vi "Insert Soak Step.vi"(0 "VISA resource name":refnum<visa-resource-name>, 1 "Current Step Number (1)":i16=1, 2 "Wait For Event Inputs (0; 0; 0; 0)":u16[](array[ring])=[0, 0, 0, 0] items=["Don't Wait", "Wait For Off", "Wait For On"], 3 "Wait For Analog Inputs (0; 0; 0)":u16[](array[ring])=[0, 0, 0] items=["Don't Wait", "Wait For Analog Input"], 4 "Analog Input Values (0.0; 0.0; 0.0)":dbl[](array[numeric])=[32.0, 32.0, 32.0] format="%.2f", 5 "error in (no error)":errorcluster {"code" format="%.0x"}, 6 "Unit Address (1)":i16=1, 7 "Event Outputs (0; 0; 0; 0; 0; 0; 0; 0)":u16[](array[ring])=[0, 0, 0, 0, 0, 0, 0, 0] items=["Off", "On"], 8 "Wait For Event (0: No)":u16(ring) items=["No", "Yes"], 9 "Time (0; 0; 1)":i16[](array[numeric])=[0, 0, 1], 10 "Channel 1 Guarantee Soak (F: Off)":bool, 11 "Channel 1 PID Set (1)":u16=1, 12 "Channel 2 Guarantee Soak (F: Off)":bool, 13 "Channel 2 PID Set (6)":u16=6) -> (14 "VISA resource name out":refnum<visa-resource-name>, 19 "error out":errorcluster {"code" format="%.0x"})   [LabVIEW 2010]
doc: "This VI inserts Soak Step."
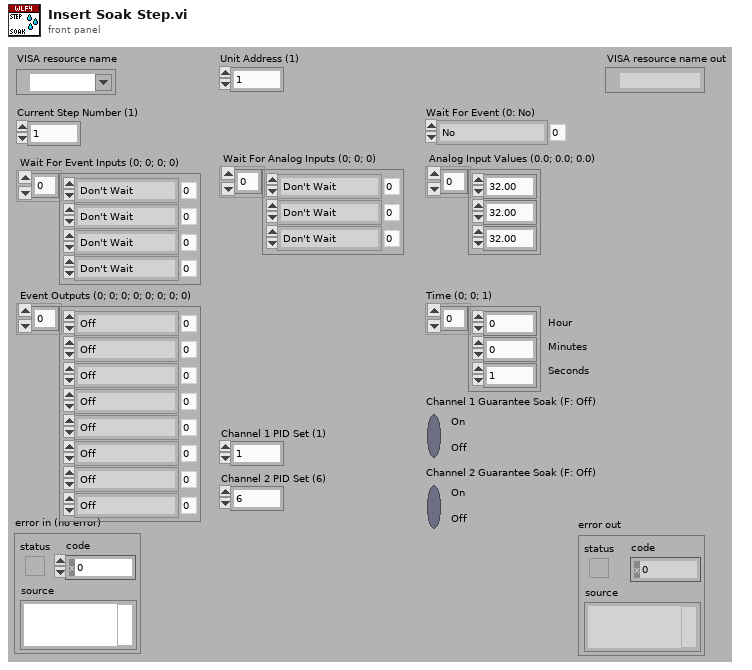
[diagram p1: front panel]
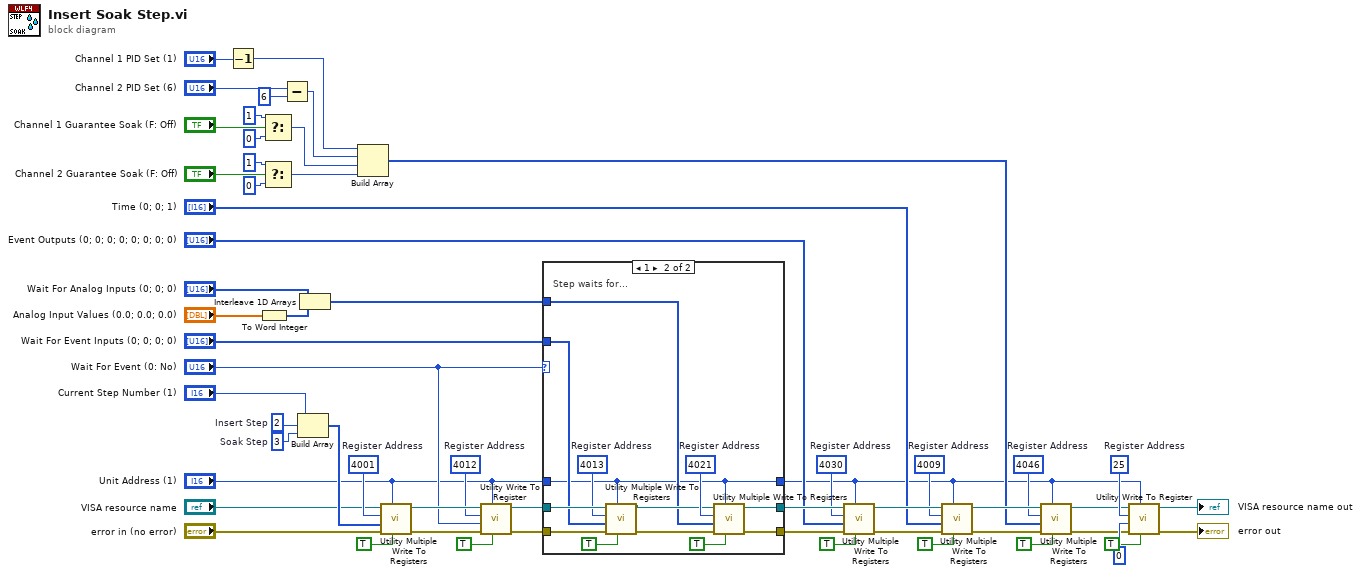
[diagram p0: block diagram]
diagram:
  w18 = u16 4046  # Register Address
  w21 = u16 4009  # Register Address
  w22 = 3  # Soak Step
  w29 = u16 25  # Register Address
  w37 = u16 4030  # Register Address
  w49 = u16 4012  # Register Address
  w55 = u16 2  # Insert Step
  w57 = u16 4001  # Register Address
  n1 = Decrement(x="Channel 1 PID Set (1)") -> (x-1=w7:u16)
  n2 = To Word Integer(number="Analog Input Values (0.0; 0.0; 0.0)") -> (16bit integer=w42:i16[])
  n3 = Select(t=1, s="Channel 1 Guarantee Soak (F: Off)", f=0) -> (s? t:f=w16:i32)
  n4 = Select(t=1, s="Channel 2 Guarantee Soak (F: Off)", f=0) -> (s? t:f=w17:i32)
  n5 = Subtract(x="Channel 2 PID Set (6)", y=u16 6) -> (x-y=w8:u16)
  n6 = Build Array("Current Step Number (1)", w55, w22) -> (w56:i32[])
  n7 = Interleave 1D Arrays("Wait For Analog Inputs (0; 0; 0)", w42) -> (w40:u16[])
  n8 = Build Array(w7, w8, w16, w17) -> (w15:i32[])
  n9 = call "Utility Multiple Write To Registers.vi"("Direct Action?"=TRUE, "Unit Address (1)"="Unit Address (1)", "error in (no error)"="error in (no error)", "Array Of Data"=w56, "Register Address (0)"=w57, "VISA resource name"="VISA resource name") -> ("error out"=w51:errorcluster, "VISA resource name out"=w50:refnum<visa-resource-name>)  [unwired: 4 in]
  n10 = call "Utility Write To Register.vi"("Direct Action?"=TRUE, "Unit Address (1)"="Unit Address (1)", "error in (no error)"=w51, "Data (0)"="Wait For Event (0: No)", "Register Address (0)"=w49, "VISA resource name"=w50) -> ("error out"=w47:errorcluster, "VISA resource name out"=w48:refnum<visa-resource-name>)  [unwired: 4 in]
  n11 = case shown="1" "Wait For Event (0: No)" {
    tunnel: w48 -> [w60 w72]
    tunnel: w47 -> [w59 w73]
    tunnel: [w59 w65] -> w39
    tunnel: [w60 w64] -> w38
    tunnel: "Unit Address (1)" -> [w58 w63]
    tunnel: [w58 w63] -> w14
    tunnel: "Wait For Event Inputs (0; 0; 0; 0)" -> [_ w70]
    tunnel: w40 -> [_ w66]
    frame 0, Default {
      # "Step does not wait"
    }
    frame 1 {
      w69 = u16 4021  # Register Address
      w71 = u16 4013  # Register Address
      # "Step waits for..."
      n12 = call "Utility Multiple Write To Registers.vi"("Direct Action?"=TRUE, "Unit Address (1)"=w63, "error in (no error)"=w73, "Array Of Data"=w70, "Register Address (0)"=w71, "VISA resource name"=w72) -> ("error out"=w68:errorcluster, "VISA resource name out"=w67:refnum<visa-resource-name>)  [unwired: 4 in]
      n13 = call "Utility Multiple Write To Registers.vi"("Direct Action?"=TRUE, "Unit Address (1)"=w63, "error in (no error)"=w68, "Array Of Data"=w66, "Register Address (0)"=w69, "VISA resource name"=w67) -> ("error out"=w65:errorcluster, "VISA resource name out"=w64:refnum<visa-resource-name>)  [unwired: 4 in]
    }
  }
  n14 = call "Utility Multiple Write To Registers.vi"("Direct Action?"=TRUE, "Unit Address (1)"=w14, "error in (no error)"=w39, "Array Of Data"="Event Outputs (0; 0; 0; 0; 0; 0; 0; 0)", "Register Address (0)"=w37, "VISA resource name"=w38) -> ("error out"=w32:errorcluster, "VISA resource name out"=w31:refnum<visa-resource-name>)  [unwired: 4 in]
  n15 = call "Utility Multiple Write To Registers.vi"("Direct Action?"=TRUE, "Unit Address (1)"=w14, "error in (no error)"=w32, "Array Of Data"="Time (0; 0; 1)", "Register Address (0)"=w21, "VISA resource name"=w31) -> ("error out"=w19:errorcluster, "VISA resource name out"=w20:refnum<visa-resource-name>)  [unwired: 4 in]
  n16 = call "Utility Multiple Write To Registers.vi"("Direct Action?"=TRUE, "Unit Address (1)"=w14, "error in (no error)"=w19, "Array Of Data"=w15, "Register Address (0)"=w18, "VISA resource name"=w20) -> ("error out"=w12:errorcluster, "VISA resource name out"=w13:refnum<visa-resource-name>)  [unwired: 4 in]
  n17 = call "Utility Write To Register.vi"("Direct Action?"=TRUE, "Unit Address (1)"=w14, "error in (no error)"=w12, "Data (0)"=i16 0, "Register Address (0)"=w29, "VISA resource name"=w13) -> ("error out"=→"error out":errorcluster, "VISA resource name out"=→"VISA resource name out":refnum<visa-resource-name>)  [unwired: 4 in]
